vi "P2-4.vi"() -> ()   [LabVIEW 2011]
panel:
  out "숫자형 2":dbl
  out "숫자형":dbl
  out "다이얼":dbl(knob) scale=0.0..10.0
  in  "노브":dbl(knob) scale=0.0..10.0
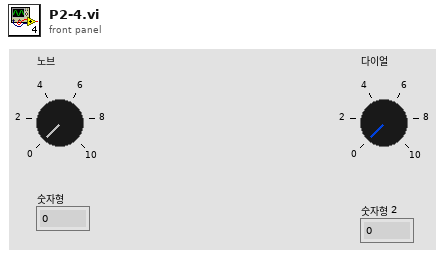
[diagram p1: front panel]
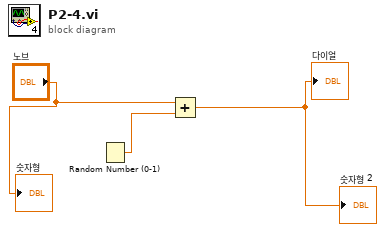
[diagram p0: block diagram]
diagram:
  n1 = Random Number (0-1)() -> (number: 0 to 1=w3:dbl)
  n2 = Add(x="노브", y=w3) -> (x+y=→"다이얼" →"숫자형 2":dbl)
  "숫자형" <- "노브"
